vi "host.vi"() -> ()   [LabVIEW 2020]
uses:
  <vilib>/Analysis/Matrix/Datatypes/RealMatrix.ctl
  <vilib>/Analysis/baseanly.llb/Real A x B.vi
  <vilib>/Analysis/7linalg.llb/Real Cholesky Factorization.vi
  <vilib>/Analysis/7linalg.llb/Real Transpose Matrix.vi
  <vilib>/Analysis/baseanly.llb/Full Cholesky Factorization.vi
  <vilib>/Analysis/baseanly.llb/Full Real Matrix Cholesky Factorization.vi
  <vilib>/FPGAPlugInAG/cRIO-9035/niLvFpga_Open_cRIO-9035.vi
  <vilib>/rvi/interface/common/dynamic/niFpgaDynamicAddResources.vi
  <vilib>/Utility/error.llb/Error Cluster From Error Code.vi
  <vilib>/rvi/errors/niLvFpgaAdjustHostInterfaceError.vi
  <vilib>/FPGAPlugInAG/Dynamic/niLvFpga_Run_Dynamic.vi
  <vilib>/Analysis/Matrix/Numeric/Subtract/Subtract - RM,RM.vi
  <vilib>/FPGAPlugInAG/Dynamic/niLvFpga_Close_Dynamic.vi
  <vilib>/rvi/interface/nirviOpenFPGA/nirviOpenFPGA.xnode
  FPGA Bitfiles/v1.1_FPGATarget_target_6xsn98Ih9FU.lvbitx
  target.vi
  <vilib>/rvi/interface/nirviMethod/nirviMethod.xnode
  <vilib>/rvi/interface/nirviCloseFPGA/nirviCloseFPGA.xnode
  <vilib>/rvi/errors/niLvFpgaMergeErrorWithErrorCode.vi
  <vilib>/Analysis/NI_AALBase.lvlib
  <vilib>/Analysis/NI_AALPro.lvlib
  <vilib>/Analysis/Matrix/NI_Matrix.lvlib
  <vilib>/FPGAPlugInAG/Dynamic/niLvFpga_WriteFifo_Dynamic.vi
  <vilib>/FPGAPlugInAG/Dynamic/niLvFpga_ReadFifo_Dynamic.vi
panel:
  out "sum of error 2":dbl
  out "error":i32
  out "L LABVIEW-FPGA":sgl[][](array[numeric])
  out "L LABVIEW":T1
  out "A input":dbl[][](array[numeric])
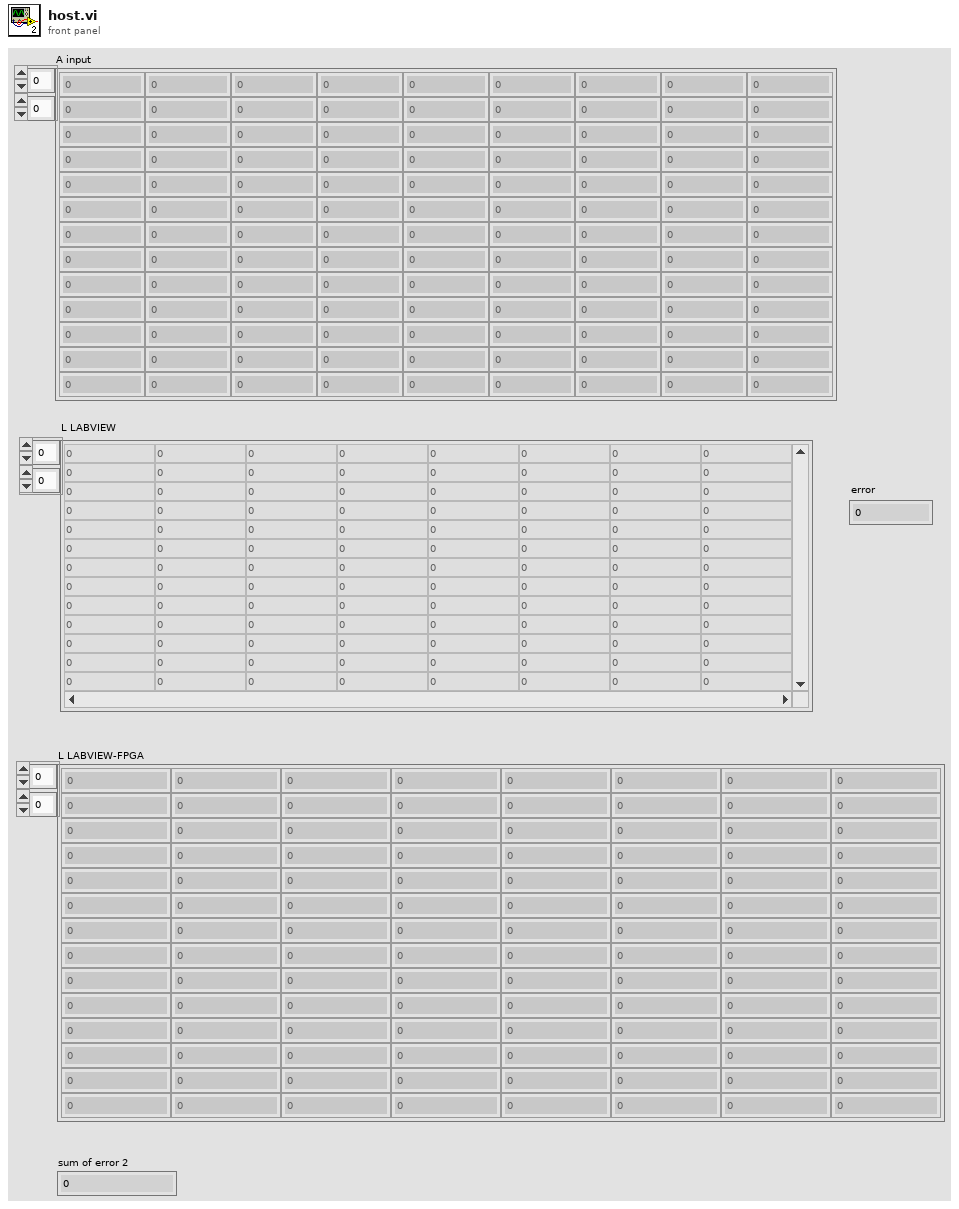
[diagram p1: front panel]
types:
  T1 = typedef "NI_Matrix.lvlib/RealMatrix.ctl" = dbl[][]
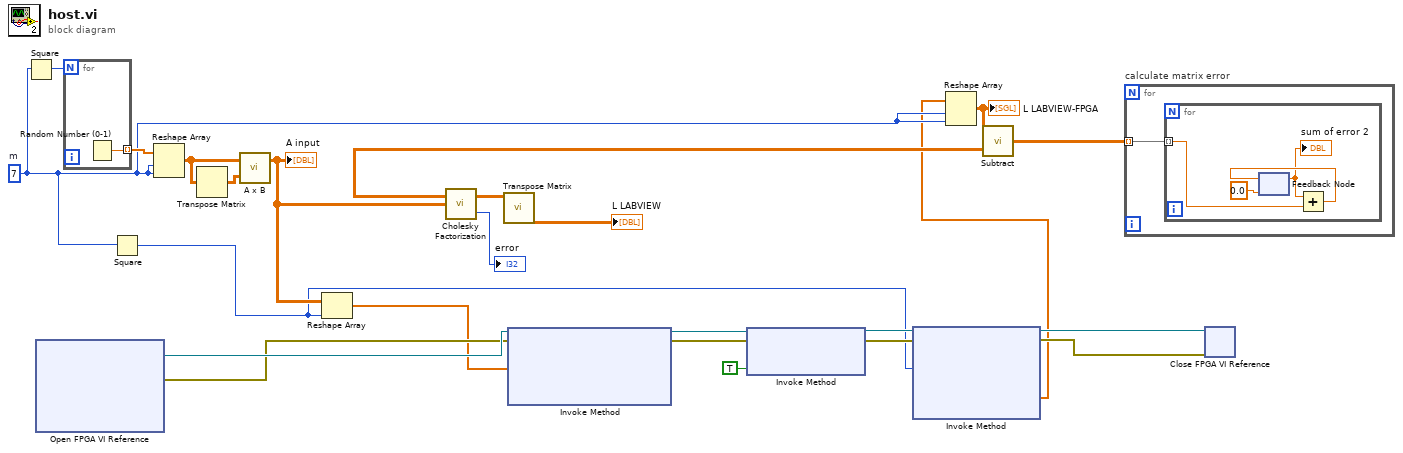
[diagram p0: block diagram]
diagram:
  w3 = 7  # m
  n1 = Square(x=w3) -> (x^2=w11:i32)
  n2 = xnode "Open FPGA VI Reference"() -> ("FPGA VI Reference Out"=w22:refnum<k20>, "error out"=w21:errorcluster)  [unwired: 2 in]
  n3 = for {
    N: w11 -> [_]
    tunnel: [w24] -> w10 mode=indexing
    n4 = Random Number (0-1)() -> (number: 0 to 1=w24:dbl)
  }
  n5 = Square(x=w3) -> (x^2=w1:i32)
  n6 = Reshape Array(w10, w3, w3) -> (w8:dbl[][])
  n7 = Transpose Matrix(1:w8) -> (0:w9:dbl[][])
  n8 = call-poly <vilib>:"A x B.vi"("B"=w9, "A"=w8) -> ("A x B"=w7:T1)  [unwired: 1 out]
  "A input" <- w7
  n9 = Reshape Array(w7, w1) -> (w4:dbl[])
  n10 = call-poly <vilib>:"Cholesky Factorization.vi"("A"=w7) -> ("Cholesky"=w15:T1, "error"=→"error":i32)
  n11 = call-poly <vilib>:"Transpose Matrix.vi"("Input Matrix"=w15) -> ("Matrix Transpose"=w12:T1)  [unwired: 9 in, 1 out]
  "L LABVIEW" <- w12
  n12 = xnode "Invoke Method"("FPGA VI Reference In"=w22, "error in"=w21, "Data"=w4) -> ("FPGA VI Reference Out"=w6:refnum<k20>, "error out"=w5:errorcluster)  [unwired: 1 in, 1 out]
  n13 = xnode "Invoke Method"("FPGA VI Reference In"=w6, "error in"=w5, "Wait Until Done (F)"=TRUE) -> ("FPGA VI Reference Out"=w20:refnum<k20>, "error out"=w19:errorcluster)
  n14 = xnode "Invoke Method"("FPGA VI Reference In"=w20, "error in"=w19, "Number of Elements"=w1) -> ("FPGA VI Reference Out"=w18:refnum<k20>, "error out"=w17:errorcluster, "Data"=w2:sgl[])  [unwired: 1 in, 1 out]
  n15 = Reshape Array(w2, w3, w3) -> (w13:sgl[][])
  "L LABVIEW-FPGA" <- w13
  n16 = call-poly <vilib>:"Subtract.vi"("Real Matrix B"=w12, "Real Matrix A"=w13) -> ("A - B"=w14:T1)
  n17 = for "calculate matrix error" {
    tunnel: w14 -> [w25] mode=indexing
    n18 = for {
      tunnel: w25 -> [w29] mode=indexing
      n19 = feedback #1(0.0) -> (w27:dbl)
      "sum of error 2" <- w27
      n20 = Add(x=w27, y=w29) -> (x+y=w28:dbl)
      n21 = feedback-in #1(w28) -> ()
    }
  }
  n22 = xnode "Close FPGA VI Reference"("FPGA VI Reference In"=w18, "error in"=w17) -> ()  [unwired: 1 out]
